vi "Format Values for String.vi"(11 "Values":string[](array[string])) -> (3 "Value String":string)   [LabVIEW 2017, in "VIs to Interface LabVIEW and MySQL dotNET Connector.lvlib"]
doc: "Convert a list of values into the correctly formatted string for use in an SQL command"
uses:
  VIs to Interface LabVIEW and MySQL dotNET Connector.lvlib
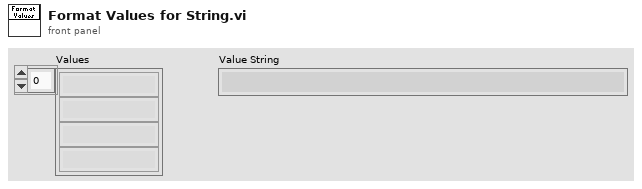
[diagram p1: front panel]
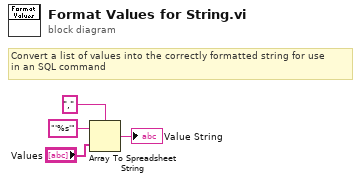
[diagram p0: block diagram]
diagram:
  # "Convert a list of values into the correctly formatted string for use\nin an SQL command"
  n1 = Array To Spreadsheet String(delimiter (Tab)=",", array="Values", 3:"'%s'" ("format string")) -> (spreadsheet string=→"Value String":string)
